vi "Modbus_Initialize.vi"(0 "IP Address":string="localhost", 5 "Port (502)":u16=502, 7 "Slave ID (255)":u8=255, 9 "Timeout (10000)":i32=10000, 11 "error in (no error)":errorcluster) -> (4 "MB_TCP session":refnum<class "MB_Master_TCP.lvclass">, 15 "error out":errorcluster)   [LabVIEW 2026]
uses:
  <vilib>/Plasmionique/MB Master/MB_Master_TCP/MB_Master_TCP.lvclass
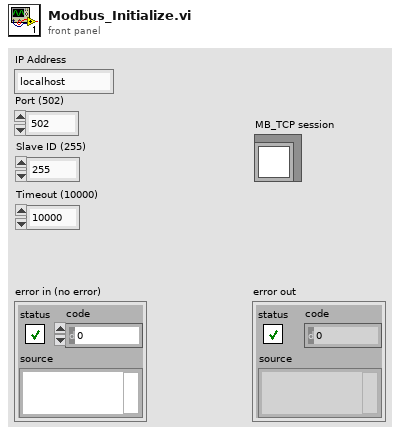
[diagram p1: front panel]
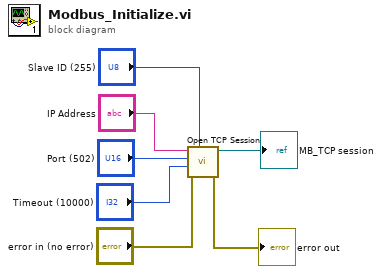
[diagram p0: block diagram]
diagram:
  n1 = call <vilib>:"Open TCP Session.vi"("Slave ID (255)"="Slave ID (255)", "error in (no error)"="error in (no error)", "Timeout (10000)"="Timeout (10000)", "Port (502)"="Port (502)", "IP Address"="IP Address") -> ("error out"=→"error out":errorcluster, "MB_TCP session"=→"MB_TCP session":refnum<class "MB_Master_TCP.lvclass">)  [unwired: 5 in]
